vi "Get Configured Audio Device ID.vi"(8 "error in (no error)":errorcluster, 11 "Audio Device Refnum In":T1) -> (0 "error out":errorcluster, 1 "Actual Device ID":u8[](array[numeric]), 2 "Configured Device ID":u8[](array[numeric]), 3 "Audio Device Refnum Out":T1)   [LabVIEW 2020, in "G-Audio.lvlib"]
doc: "Get information about the configured audio device."
uses:
  G-Audio.lvlib
  Controls/Audio Device Refnum.ctl
  <vilib>/Utility/error.llb/Error Cluster From Error Code.vi
  lib/g_audio_32.dll
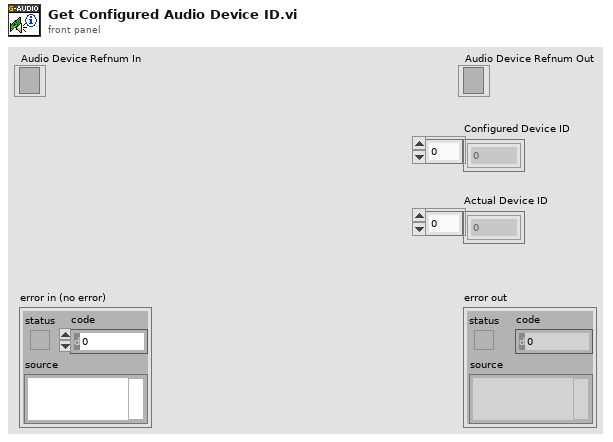
[diagram p1: front panel]
types:
  T1 = typedef "G-Audio.lvlib/Audio Device Refnum.ctl" = refnum<file>
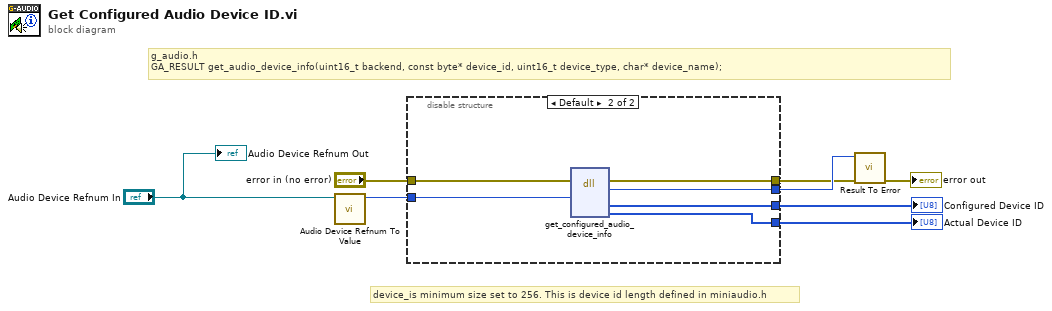
[diagram p0: block diagram]
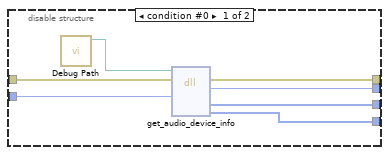
[diagram p2: hidden frame]
diagram:
  # "device_is minimum size set to 256. This is device id length defined in miniaudio.h"
  # "g_audio.h\nGA_RESULT get_audio_device_info(uint16_t backend, const byte* device_id, uint16_t device_type, char* device_name);"
  n1 = call "Audio Device Refnum To Value.vi"("Audio Device Refnum"="Audio Device Refnum In") -> ("Refnum Value"=w3:i32)  [unwired: 10 in]
  n2 = disable-structure shown="Default" {
    disable-tunnel: "error in (no error)" -> [w15 w21]
    disable-tunnel: [w13 w19] -> w7
    disable-tunnel: [w14 w20] -> w6
    disable-tunnel: w3 -> [w11 w18]
    disable-tunnel: [w10 w17] -> w2
    disable-tunnel: [w9 w16] -> w1
    frame condition #0 {
      n3 = call "Debug Path.vi"() -> ("Debug Path"=w12:path)  [unwired: 11 in]
      n4 = dll-call lib="?" fn="get_audio_device_info"(path in=w12, error in=w15, "refnum"=w11) -> (error out=w14:errorcluster, "result"=w13:i32, "config_device_id"=w10:u8[], "actual_device_id"=w9:u8[])  [unwired: 4 in, 1 out]
    }
    frame condition #1 (active) {
      n5 = dll-call lib="C:/github/dataflowg/g-audio/src/LabVIEW/G-Audio/lib/g_audio_*.*" fn="get_configured_audio_device_info"(error in=w21, "refnum"=w18) -> (error out=w20:errorcluster, "result"=w19:i32, "config_device_id"=w17:u8[], "actual_device_id"=w16:u8[])  [unwired: 5 in, 1 out]
    }
  }
  "Actual Device ID" <- w1
  "Configured Device ID" <- w2
  n6 = call "Result To Error.vi"("error in (no error)"=w6, "Result Code"=w7) -> ("error out"=→"error out":errorcluster)  [unwired: 9 in]
  "Audio Device Refnum Out" <- "Audio Device Refnum In"
